vi "Global Variables.vi"() -> ()   [LabVIEW 2017]
panel:
  out "Speed":dbl
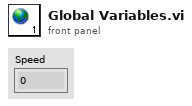
[diagram p1: front panel]
diagram:
